vi "RemoveObject.vi"(0 "__args":cluster{"targetVi":string, "objectRef":i32}) -> (1 "__return":i32, 2 "__errStatus":bool, 3 "__errCode":i32, 4 "__errSource":string)   [LabVIEW 2013]
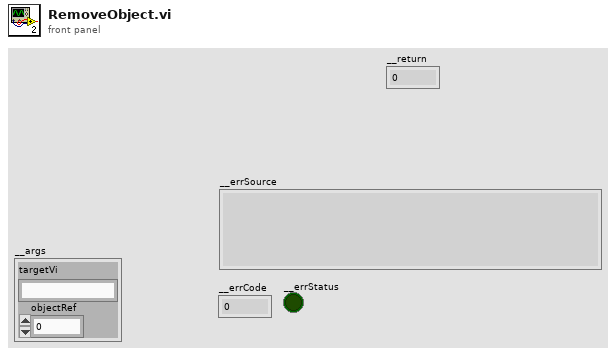
[diagram p1: front panel]
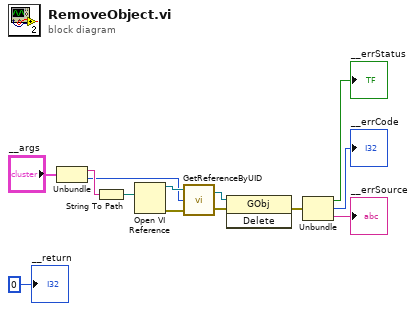
[diagram p0: block diagram]
diagram:
  n1 = Unbundle("__args") -> ("targetVi"=w9:string, "objectRef"=w5:i32)
  n2 = String To Path(string=w9) -> (path=w8:path)
  n3 = Open VI Reference(vi path=w8) -> (vi reference=w6:refnum<vi>, error out=w3:errorcluster)  [unwired: 5 in]
  n4 = call "GetReferenceByUID.vi"("error in (no error)"=w3, "UID"=w5, "targetVI"=w6) -> ("error out"=w2:errorcluster, "refNum"=w4:refnum<vi>)
  n5 = invoke class="GObj" method="Delete"(reference=w4, error in=w2) -> (error out=w1:errorcluster)  [unwired: 1 in, 2 out]
  n6 = Unbundle(w1) -> ("status"=→"__errStatus":bool, "code"=→"__errCode":i32, "source"=→"__errSource":string)
  "__return" <- 0
